vi "Position_Read(POS).vi"(7 "baud rate (9600)":u32=115200 caption="보 전송속도(9600)", 8 "Port":refnum<visa-resource-name>="COM4" caption="VISA 리소스 이름") -> (0 "Error Out":errorcluster caption="에러 출력", 1 "Position(Y)":i32, 2 "Position(X)":i32, 3 "VISA out":refnum<visa-resource-name>, 4 "버퍼 읽기":string)   [LabVIEW 2016]
uses:
  <vilib>/Instr/_visa.llb/VISA Flush IO Buffer Mask.ctl
  <vilib>/Instr/_visa.llb/VISA Configure Serial Port (Instr).vi
panel:
  out "부분 문자열":string
  out "Commend Count":u32
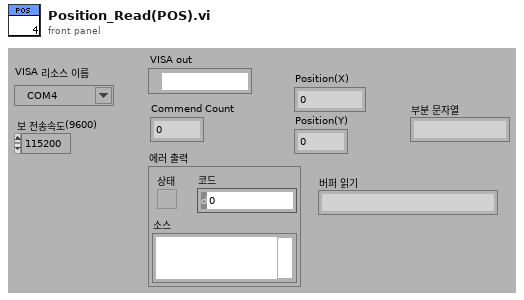
[diagram p1: front panel]
types:
  T1 = typedef "VISA Flush IO Buffer Mask.ctl" = u16
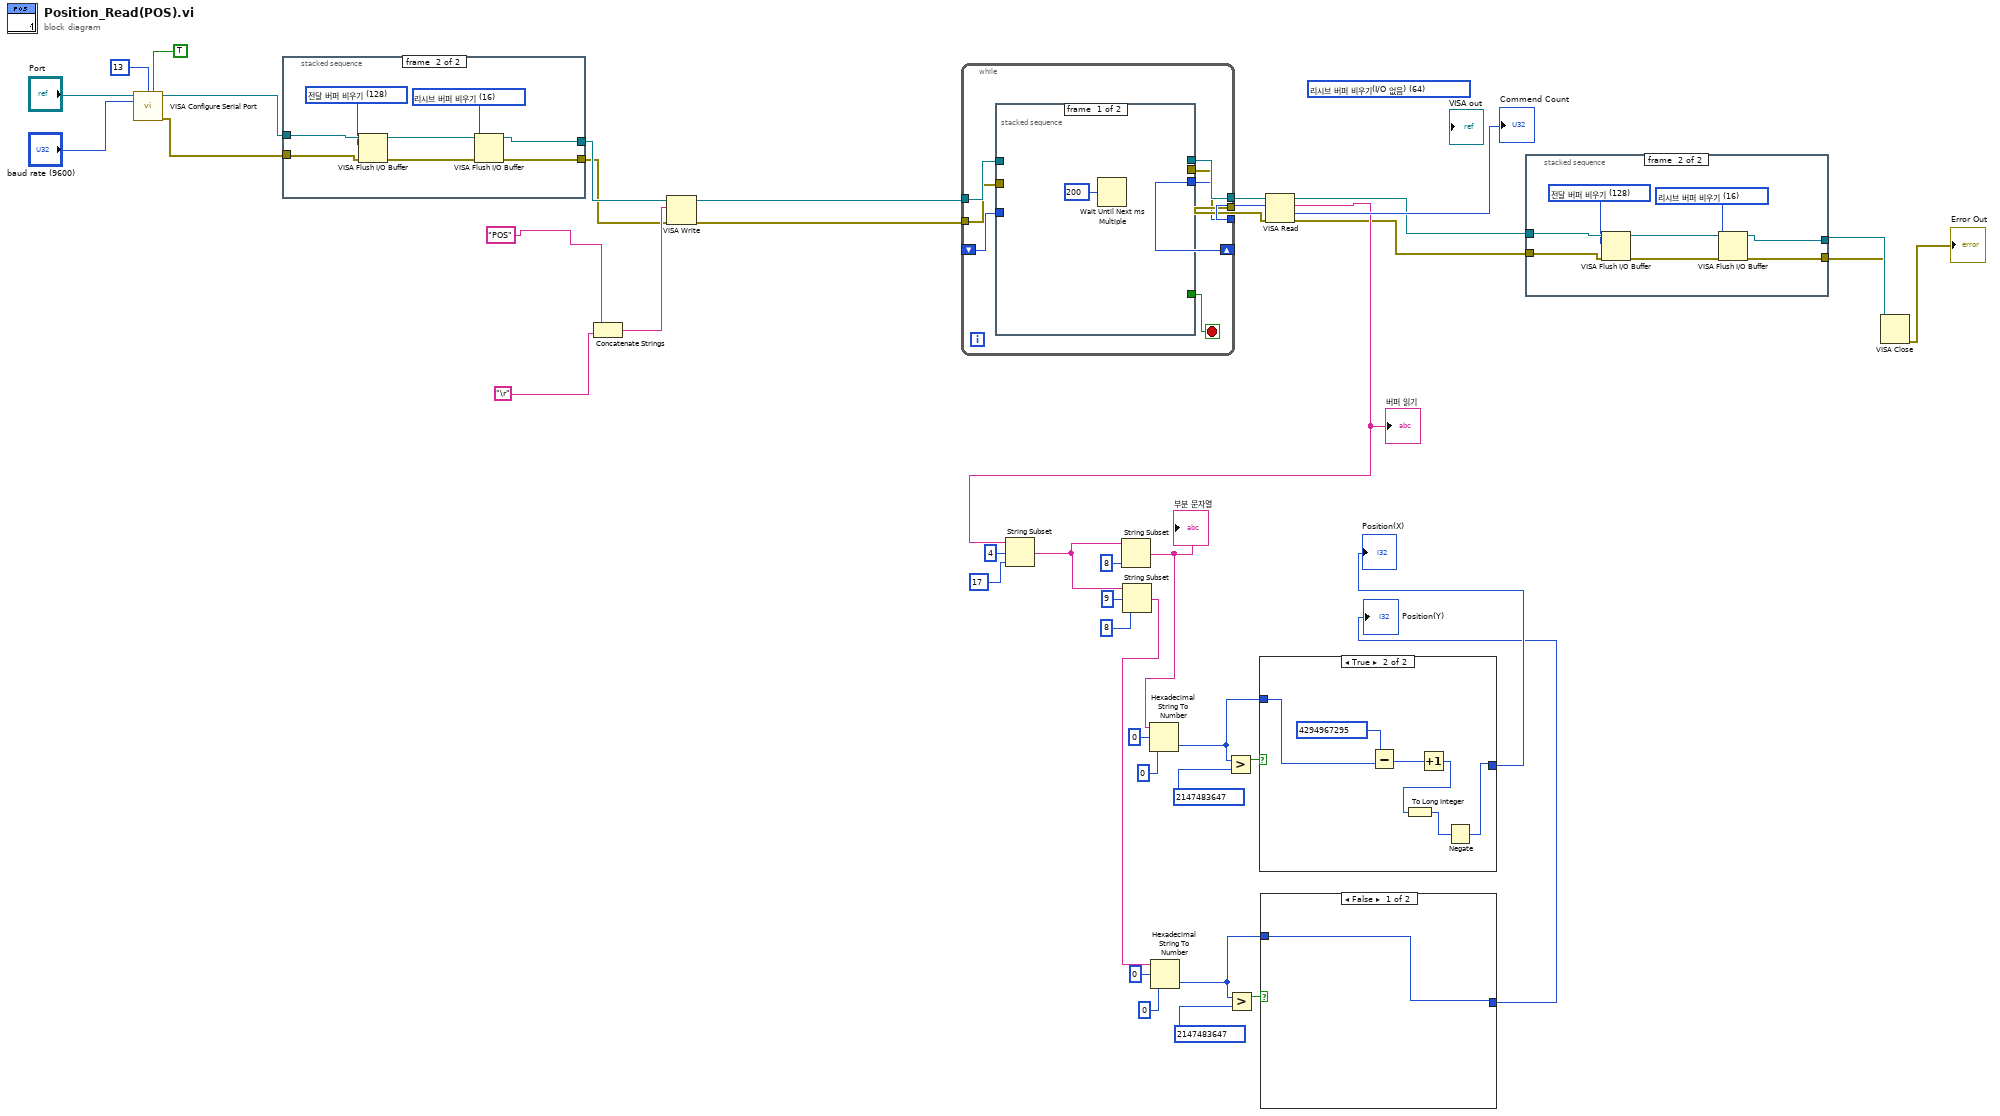
[diagram p0: block diagram]
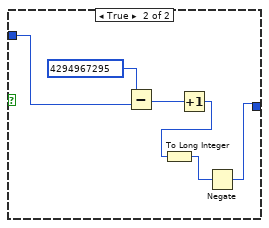
[diagram p2: hidden frame]
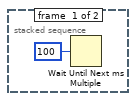
[diagram p4: hidden frame]
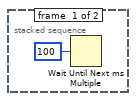
[diagram p5: hidden frame]
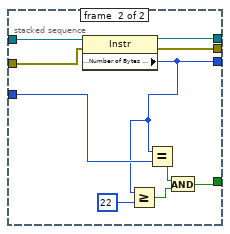
[diagram p6: hidden frame]
diagram:
  (unwired) T1 64 items=["리시브 버퍼 비우기"=16, "전달 버퍼 디바이스에 쓰기"=32, "리시브 버퍼 비우기(I/O 없음)"=64, "전달 버퍼 비우기"=128] ("Mask")
  n1 = call-poly "VISA Configure Serial Port"("VISA resource name"="Port", "termination char\n(0xA = '\\n' = LF)"=i16 13 ("termination char\n(0xA = '\\n' = LF)"), "Enable Termination\nChar (T)"=TRUE ("Enable Termination\nChar (T)"), "baud rate (9600)"="baud rate (9600)") -> ("VISA resource name out"=w22:refnum<visa-resource-name>, "error out"=w21:errorcluster)  [unwired: 10 in]
  n2 = stacked-sequence {
    tunnel: w22 -> [_ w52]
    tunnel: w21 -> [_ w51]
    tunnel: [_ w47] -> w20
    tunnel: [_ w46] -> w19
    frame #0 {
      n3 = Wait Until Next ms Multiple(millisecond multiple=u32 100 ("ms 배수")) -> ()  [unwired: 1 out]
    }
    frame #1 {
      w45 = T1 16 items=["리시브 버퍼 비우기"=16, "전달 버퍼 디바이스에 쓰기"=32, "리시브 버퍼 비우기(I/O 없음)"=64, "전달 버퍼 비우기"=128] ("Mask")
      w50 = T1 128 items=["리시브 버퍼 비우기"=16, "전달 버퍼 디바이스에 쓰기"=32, "리시브 버퍼 비우기(I/O 없음)"=64, "전달 버퍼 비우기"=128] ("Mask")
      n4 = VISA Flush I/O Buffer(VISA resource name=w52, mask (16)=w50, error in (no error)=w51) -> (VISA resource name out=w49:refnum<visa-resource-name>, error out=w48:errorcluster)
      n5 = VISA Flush I/O Buffer(VISA resource name=w49, mask (16)=w45, error in (no error)=w48) -> (VISA resource name out=w47:refnum<visa-resource-name>, error out=w46:errorcluster)
    }
  }
  n6 = Concatenate Strings("POS", "\r") -> (w31:string)
  n7 = VISA Write(VISA resource name=w20, write buffer=w31, error in (no error)=w19) -> (VISA resource name out=w29:refnum<visa-resource-name>, error out=w28:errorcluster)  [unwired: 1 out]
  n8 = while {
    tunnel: w29 -> [w59]
    tunnel: w28 -> [w58]
    tunnel: [w57] -> w43
    tunnel: [w54] -> w42
    tunnel: [w56] -> w41
    shift-right: [w54] -> _
    shift-left: _ -> [w53]
    stop <- w55 stop-if-true
    n9 = stacked-sequence {
      tunnel: w59 -> [_ w70]
      tunnel: w58 -> [_ w69]
      tunnel: [_ w68] -> w57
      tunnel: [_ w67] -> w56
      tunnel: [_ w61] -> w55
      tunnel: [_ w65] -> w54
      tunnel: w53 -> [_ w66]
      frame #0 {
        n10 = Wait Until Next ms Multiple(millisecond multiple=u32 200 ("ms 배수")) -> ()  [unwired: 1 out]
      }
      frame #1 {
        n11 = property class="Instr"(reference=w70, error in=w69) -> (reference out=w68:refnum<visa-resource-name>, error out=w67:errorcluster, "Serial Settings:Number of Bytes at Serial Port"=w65:u32)
        n12 = Greater Or Equal?(x=w65, y=u32 22) -> (x >= y?=w62:bool)
        n13 = Equal?(x=w65, y=w66) -> (x = y?=w63:bool)
        n14 = And(x=w63, y=w62) -> (x .and. y?=w61:bool)
      }
    }
  }
  n15 = VISA Read(VISA resource name=w43, byte count=w42, error in (no error)=w41) -> (VISA resource name out=w18:refnum<visa-resource-name>, read buffer=w39:string, return count=→"Commend Count":u32, error out=w17:errorcluster)
  "버퍼 읽기" <- w39
  n16 = String Subset(string=w39, offset (0)=4 ("오프셋(0)"), length (rest)=17 ("길이(나머지)")) -> (substring=w36:string)
  n17 = String Subset(string=w36, length (rest)=8 ("길이(나머지)")) -> (substring=w9:string)  [unwired: 1 in]
  "부분 문자열" <- w9
  n18 = String Subset(string=w36, offset (0)=9 ("오프셋(0)"), length (rest)=8 ("길이(나머지)")) -> (substring=w2:string)
  n19 = Hexadecimal String To Number(string=w9, offset=0 ("오프셋"), default (0uL)=0 ("기본(0 U32)")) -> (number=w10:i32)  [unwired: 1 out]
  n20 = Hexadecimal String To Number(string=w2, offset=0 ("오프셋"), default (0uL)=0 ("기본(0 U32)")) -> (number=w3:i32)  [unwired: 1 out]
  n21 = Greater?(x=w10, y=2147483647) -> (0:w11:bool)
  n22 = Greater?(x=w3, y=2147483647) -> (0:w4:bool)
  n23 = case shown="True" w11 {
    tunnel: w10 -> [w71 w76]
    tunnel: [w71 w72] -> w8
    frame False {
    }
    frame True {
      n24 = Subtract(x=u32 4294967295, y=w76) -> (x-y=w75:u32)
      n25 = Increment(x=w75) -> (x+1=w73:u32)
      n26 = To Long Integer(number=w73) -> (32bit integer=w74:i32)
      n27 = Negate(x=w74) -> (-x=w72:i32)
    }
  }
  "Position(X)" <- w8
  n28 = case shown="False" w4 {
    tunnel: w3 -> [w78 w83]
    tunnel: [w78 w79] -> w1
    frame False {
    }
    frame True {
      n29 = Subtract(x=u32 4294967295, y=w83) -> (x-y=w82:u32)
      n30 = Increment(x=w82) -> (x+1=w80:u32)
      n31 = To Long Integer(number=w80) -> (32bit integer=w81:i32)
      n32 = Negate(x=w81) -> (-x=w79:i32)
    }
  }
  "Position(Y)" <- w1
  n33 = stacked-sequence {
    tunnel: w18 -> [_ w93]
    tunnel: w17 -> [_ w92]
    tunnel: [_ w88] -> w16
    tunnel: [_ w87] -> w15
    frame #0 {
      n34 = Wait Until Next ms Multiple(millisecond multiple=u32 100 ("ms 배수")) -> ()  [unwired: 1 out]
    }
    frame #1 {
      w86 = T1 16 items=["리시브 버퍼 비우기"=16, "전달 버퍼 디바이스에 쓰기"=32, "리시브 버퍼 비우기(I/O 없음)"=64, "전달 버퍼 비우기"=128] ("Mask")
      w91 = T1 128 items=["리시브 버퍼 비우기"=16, "전달 버퍼 디바이스에 쓰기"=32, "리시브 버퍼 비우기(I/O 없음)"=64, "전달 버퍼 비우기"=128] ("Mask")
      n35 = VISA Flush I/O Buffer(VISA resource name=w93, mask (16)=w91, error in (no error)=w92) -> (VISA resource name out=w90:refnum<visa-resource-name>, error out=w89:errorcluster)
      n36 = VISA Flush I/O Buffer(VISA resource name=w90, mask (16)=w86, error in (no error)=w89) -> (VISA resource name out=w88:refnum<visa-resource-name>, error out=w87:errorcluster)
    }
  }
  n37 = VISA Close(VISA resource name=w16, error in (no error)=w15) -> (error out=→"Error Out":errorcluster)
